vi "5492_AutoGrab.vi"   [LabVIEW 2017]
uses:
  5492_CollectButtons.vi
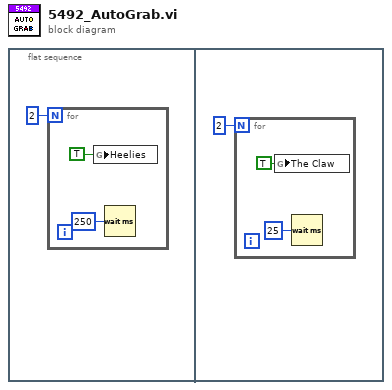
[diagram p0: block diagram]
diagram:
  n1 = flat-sequence {
    frame #0 {
      n2 = for {
        N: 2 -> [_]
        n3 = global write "5492_CollectButtons.vi" "Heelies"(TRUE ("Heelies")) -> ()
        n4 = Wait (ms)(milliseconds to wait=u32 250) -> ()  [unwired: 1 out]
      }
    }
    frame #1 {
      n5 = for {
        N: 2 -> [_]
        n6 = global write "5492_CollectButtons.vi" "The Claw"(TRUE ("Heelies")) -> ()
        n7 = Wait (ms)(milliseconds to wait=u32 25) -> ()  [unwired: 1 out]
      }
    }
  }
